vi "HardStopCurrentProcess (SubVI).vi"(11 "VISA Refnum in":refnum<visa-resource-name>) -> ()   [LabVIEW 2020]
uses:
  <vilib>/Instr/_visa.llb/VISA Configure Serial Port (Instr).vi
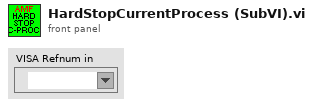
[diagram p1: front panel]
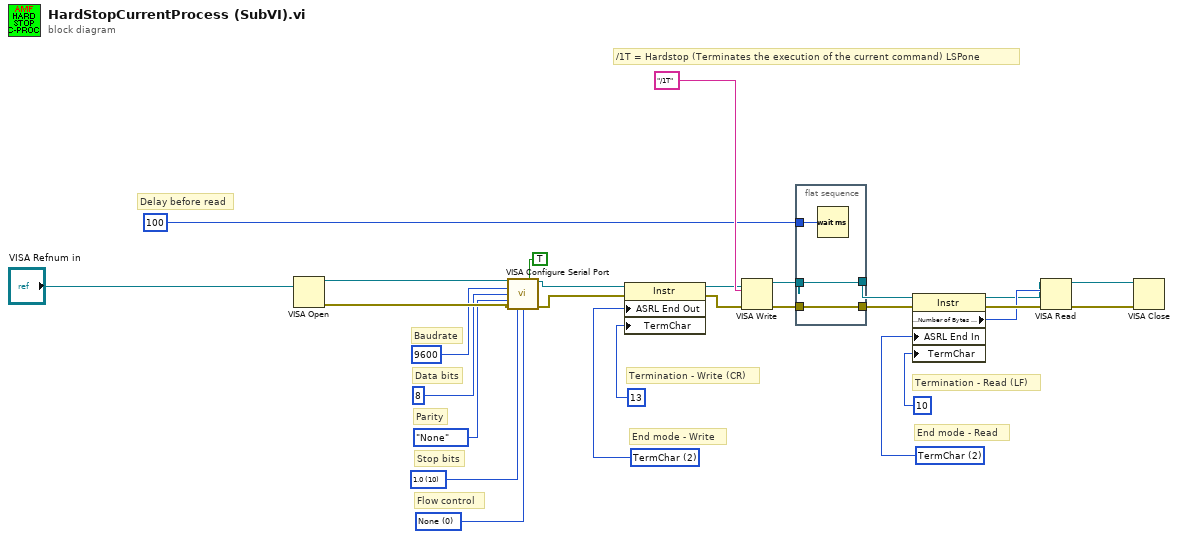
[diagram p0: block diagram]
diagram:
  w1 = u16 2 items=["None", "Last Bit", "TermChar"] ("Serial Settings:End Mode for Reads")
  w4 = u16 2 items=["None", "Last Bit", "TermChar", "Break"] ("Serial Settings:End Mode for Writes")
  w5 = u16 0 items=["None", "XON/XOFF", "RTS/CTS", "XON/XOFF & RTS/CTS", "DTR/DSR", "XON/XOFF & DTR/DSR"] ("flow control (0:none)")
  w6 = u16 10 items=["1.0"=10, "1.5"=15, "2.0"=20] ("stop bits (10: 1 bit)")
  # "/1T = Hardstop (Terminates the execution of the current command) LSPone"
  # "End mode - Read"
  # "Termination - Read (LF)"
  # "End mode - Write"
  # "Termination - Write (CR)"
  # "Flow control"
  # "Stop bits"
  # "Parity"
  # "Data bits"
  # "Baudrate"
  # "Delay before read"
  n1 = VISA Open(VISA resource name="VISA Refnum in") -> (VISA resource name=w14:refnum<visa-resource-name>, error out=w13:errorcluster)  [unwired: 4 in]
  n2 = call-poly "VISA Configure Serial Port"("VISA resource name"=w14, "Enable Termination\nChar (T)"=TRUE, "baud rate (9600)"=u32 9600, "data bits (8)"=u16 8, "parity (0:none)"=enum16{"None", "Odd", "Even", "Mark", "Space"}."None", "error in (no error)"=w13, "stop bits (10: 1 bit)"=w6, "flow control (0:none)"=w5) -> ("VISA resource name out"=w21:refnum<visa-resource-name>, "error out"=w20:errorcluster)  [unwired: 1 in, 5 out]
  n3 = property class="Instr"(reference=w21, error in=w20, "ASRL End Out"=w4, "TermChar"=u8 13 ("Message Based Settings:Termination Character")) -> (reference out=w19:refnum<visa-resource-name>, error out=w18:errorcluster)
  n4 = VISA Write(VISA resource name=w19, write buffer="/1T", error in (no error)=w18) -> (VISA resource name out=w25:refnum<visa-resource-name>, error out=w27:errorcluster)  [unwired: 1 out]
  n5 = flat-sequence {
    tunnel: w27 -> [w30]
    tunnel: [w30] -> w26
    tunnel: w25 -> [w29]
    tunnel: [w29] -> w10
    tunnel: u32 100 ("delay before read (ms)") -> [w31]
    frame #0 {
      n6 = Wait (ms)(milliseconds to wait=w31) -> ()  [unwired: 1 out]
    }
  }
  n7 = property class="Instr"(reference=w10, error in=w26, "ASRL End In"=w1, "TermChar"=u8 10 ("Message Based Settings:Termination Character")) -> (reference out=w11:refnum<visa-resource-name>, error out=w23:errorcluster, "Serial Settings:Number of Bytes at Serial Port"=w22:u32)
  n8 = VISA Read(VISA resource name=w11, byte count=w22, error in (no error)=w23) -> (VISA resource name out=w16:refnum<visa-resource-name>, error out=w15:errorcluster)  [unwired: 2 out]
  n9 = VISA Close(VISA resource name=w16, error in (no error)=w15) -> ()  [unwired: 1 out]
